vi "compass_lines.vi"(4 "center":cluster{"x":i32, "y":i32}={"x"=37, "y"=37}, 5 "color":u32(colorbox)=16448250, 6 "size":i32=37, 7 "angle":i32, 10 "pict in":picture) -> (3 "pict out":picture)   [LabVIEW 2017]
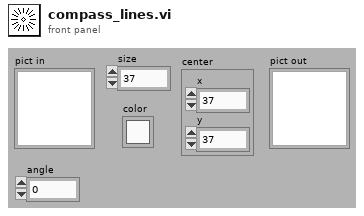
[diagram p1: front panel]
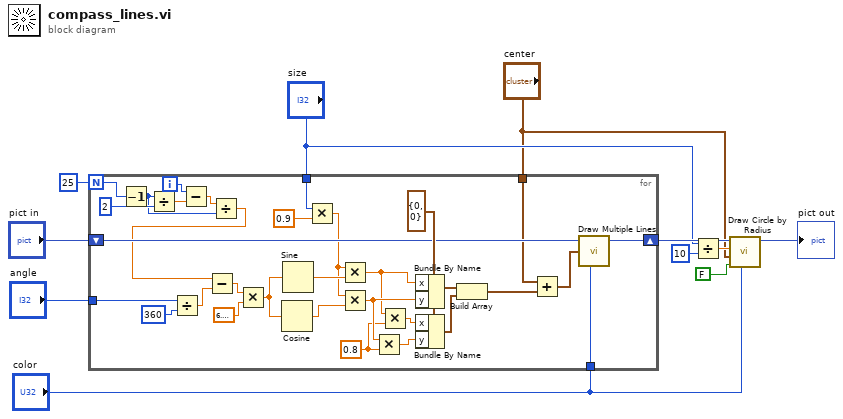
[diagram p0: block diagram]
diagram:
  n1 = for {
    N: 25 ("Numeric") -> [w40]
    tunnel: "size" -> [w21]
    shift-right: [w25] -> w8
    shift-left: "pict in" -> [w24]
    tunnel: "center" -> [w22]
    tunnel: "angle" -> [w15]
    tunnel: "color" -> [w12]
    i -> [w39]
    w27 = 0.8 ("y")
    w26 = cluster{"x":i16, "y":i16} {"x"=0, "y"=0}
    n2 = Decrement(x=w40) -> (x-1=w41:i32)
    n3 = Divide(x=w41, y=2) -> (x/y=w42:dbl)
    n4 = Divide(x=w15, y=360) -> (x/y=w13:dbl)
    n5 = Subtract(x=w39, y=w42) -> (x-y=w38:dbl)
    n6 = Divide(x=w38, y=w41) -> (x/y=w16:dbl)
    n7 = Subtract(x=w16, y=w13) -> (x-y=w17:dbl)
    n8 = Multiply(x=w17, y=6.283185307179586) -> (x*y=w18:dbl)
    n9 = Cosine(x=w18) -> (cos(x)=w33:dbl)
    n10 = Sine(x=w18) -> (sin(x)=w34:dbl)
    n11 = Multiply(x=w21, y=0.9) -> (x*y=w20:dbl)
    n12 = Multiply(x=w20, y=w34) -> (x*y=w28:dbl)
    n13 = Multiply(x=w20, y=w33) -> (x*y=w32:dbl)
    n14 = Multiply(x=w32, y=w27) -> (x*y=w30:dbl)
    n15 = Multiply(x=w28, y=w27) -> (x*y=w29:dbl)
    n16 = Bundle By Name(cluster=w26, "x"=w28, "y"=w32) -> (w35:cluster{"x":i16, "y":i16})
    n17 = Bundle By Name(cluster=w26, "x"=w29, "y"=w30) -> (w31:cluster{"x":i16, "y":i16})
    n18 = Build Array(w35, w31) -> (w36:cluster{"x":i16, "y":i16}[])
    n19 = Add(x=w22, y=w36) -> (x+y=w23:cluster{"x":i32, "y":i32}[])
    n20 = call <vilib>:"Draw Multiple Lines.vi"("picture"=w24, "line endpoints"=w23, "color(black)"=w12) -> ("new picture"=w25:picture)  [unwired: 6 in]
  }
  n21 = Divide(x="size", y=10) -> (x/y=w4:dbl)
  n22 = call <vilib>:"Draw Circle by Radius.vi"("color(black)"="color", "fill?(F)"=FALSE, "pixel center"="center", "radius"=w4, "picture"=w8) -> ("new picture"=→"pict out":picture)  [unwired: 6 in]
